vi "Create Child Class Override VIs.vi"(8 "error in":errorcluster, 10 "Service Impl class in":refnum<vi>, 11 "base class dynamic member VIs":refnum<vi>[](array[refnum])=[refnum]) -> (0 "error out":errorcluster, 3 "Service Impl class out":refnum<vi>)   [LabVIEW 2019, in "gRPC Template Creation Utility.lvlib"]
uses:
  gRPC Template Creation Utility.lvlib
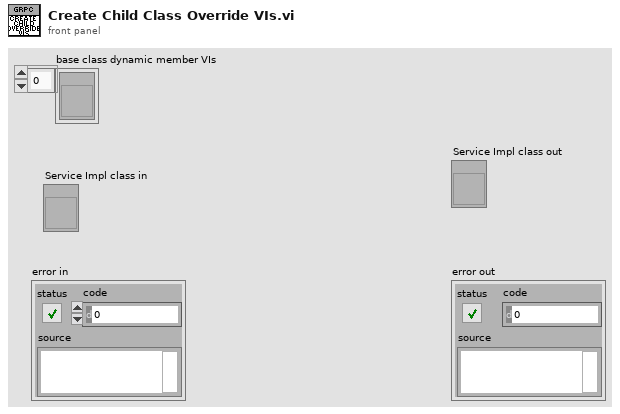
[diagram p1: front panel]
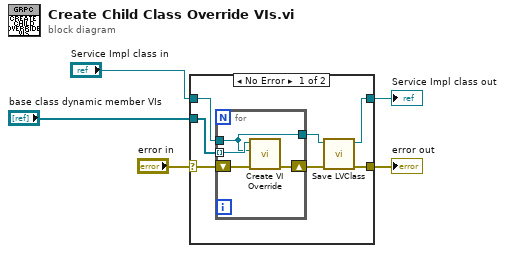
[diagram p0: block diagram]
diagram:
  n1 = case shown="No Error" "error in" {
    selector: "error in" -> [w12 w18]
    tunnel: [w7 w18] -> w4
    tunnel: "base class dynamic member VIs" -> [w11 _]
    tunnel: "Service Impl class in" -> [w10 w17]
    tunnel: [w6 w17] -> w1
    frame No Error {
      n2 = for {
        shift-right: [w14] -> w8
        shift-left: w12 -> [w15]
        tunnel: w11 -> [w16] mode=indexing
        tunnel: w10 -> [w13]
        tunnel: [w13] -> w9
        n3 = call "Create VI Override.vi"("error in (no error)"=w15, "Child class in"=w13, "Parent Method VI in"=w16) -> ("error out"=w14:errorcluster)  [unwired: 6 in, 2 out]
      }
      n4 = call "Save LVClass.vi"("error in (no error)"=w8, "LVClassLibrary in"=w9) -> ("error out"=w7:errorcluster, "LVClassLibrary out"=w6:refnum<vi>)  [unwired: 8 in]
    }
    frame Error {
    }
  }
  "error out" <- w4
  "Service Impl class out" <- w1
